vi "CreateCString.vi"() -> ()   [LabVIEW 2022 SP3]
uses:
  <vilib>/Utility/file.llb/Read From Spreadsheet File (I64).vi
panel:
  out "string":string
  in  "Path":path
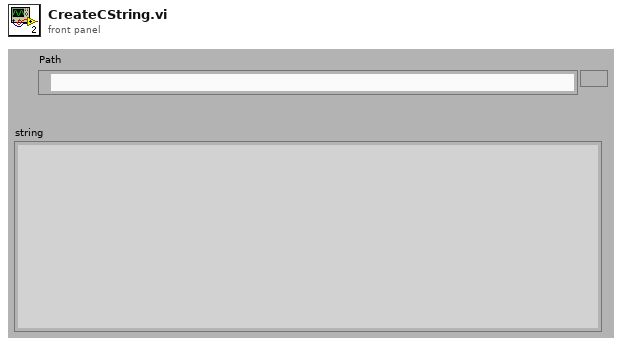
[diagram p1: front panel]
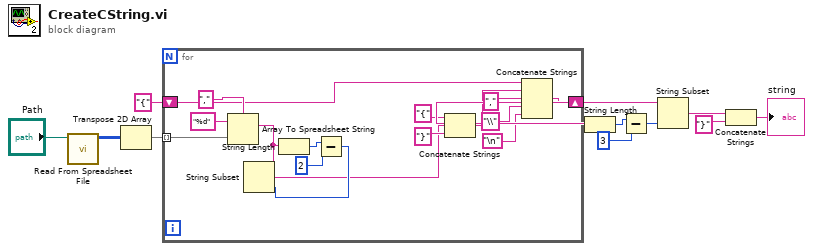
[diagram p0: block diagram]
diagram:
  n1 = call-poly <vilib>:"Read From Spreadsheet File.vi"("file path (dialog if empty)"="Path") -> ("all rows"=w10:i64[][])  [unwired: 6 in, 4 out]
  n2 = Transpose 2D Array(2D array=w10) -> (transposed array=w9:i64[][])
  n3 = for {
    tunnel: w9 -> [w27] mode=indexing
    shift-right: [w20] -> w7
    shift-left: "{" ("string") -> [w22]
    n4 = Array To Spreadsheet String(delimiter (Tab)=",", array=w27, 3:"%d" ("format string")) -> (spreadsheet string=w16:string)
    n5 = String Length(string=w16) -> (length=w13:i32)
    n6 = Subtract(x=w13, y=2) -> (x-y=w15:i32)
    n7 = String Subset(string=w16, length (rest)=w15) -> (substring=w14:string)  [unwired: 1 in]
    n8 = Concatenate Strings("{" ("string"), w14, "}" ("string")) -> (w21:string)
    n9 = Concatenate Strings(w22, w21, "," ("string"), "\\" ("string"), "\n") -> (w20:string)
  }
  n10 = String Length(string=w7) -> (length=w2:i32)
  n11 = Subtract(x=w2, y=3) -> (x-y=w6:i32)
  n12 = String Subset(string=w7, length (rest)=w6) -> (substring=w5:string)  [unwired: 1 in]
  n13 = Concatenate Strings(w5, "}" ("string")) -> (→"string":string)
